vi "Choreo_Choreo_LoadTrajectoryTypeString.vi"(11 "trajectoryJsonString":string) -> (0 "Error":bool, 3 "TrajectoryType":T1)   [LabVIEW 2019, in "ChoreoLib.lvlib"]
doc: "Parse a choreo trajectory from a JSON formatted string to determine the type of trajectory, differential or swerve.. \n\nInputs: \n - trajectoryJsonString - string- The string containing the choreo trajectory. These are actually internally formatted as JSON files.\n\nOutputs:\n - TrajectoryType - enum - Type of trajectory found in the file.\n - Error out - cluster - Error cluster"
uses:
  ChoreoLib.lvlib
  ENum/Choreo_Util_TrajectoryType.ctl
panel:
  out "sampleType":string
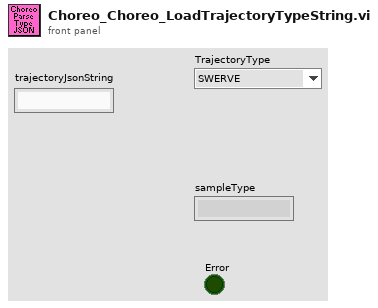
[diagram p1: front panel]
types:
  T1 = typedef "ChoreoLib.lvlib/Choreo_Util_TrajectoryType.ctl" = enum16{"SWERVE", "DIFFERENTIAL", "UNKNOWN"}
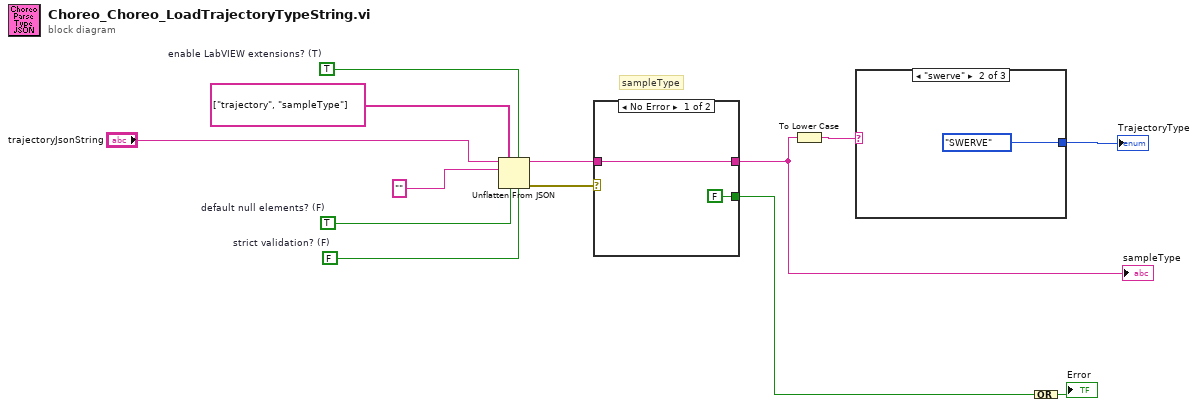
[diagram p0: block diagram]
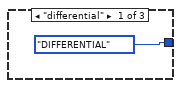
[diagram p2: hidden frame]
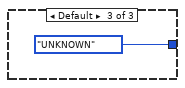
[diagram p3: hidden frame]
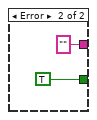
[diagram p4: hidden frame]
diagram:
  w9 = FALSE  # strict validation? (F)
  w10 = TRUE  # default null elements? (F)
  w11 = TRUE  # enable LabVIEW extensions? (T)
  # "sampleType"
  n1 = Unflatten From JSON(path=string[] ["trajectory", "sampleType"] ("path 7"), enable LabVIEW extensions? (T)=w11, JSON string="trajectoryJsonString", type and defaults="", default null elements? (F)=w10, strict validation? (F)=w9) -> (value=w12:string, error out=w13:errorcluster)  [unwired: 1 in]
  n2 = case shown="No Error" w13 {
    tunnel: w12 -> [w14 _]
    tunnel: [FALSE TRUE] -> w5
    tunnel: [w14 ""] -> w2
    frame No Error {
    }
    frame Error {
    }
  }
  "sampleType" <- w2
  n3 = To Lower Case(string=w2) -> (all lower case string=w3:string)
  n4 = case shown="\"swerve\"" w3 {
    tunnel: [Choreo_Util_TrajectoryType."DIFFERENTIAL" ("TrajectoryType") Choreo_Util_TrajectoryType."SWERVE" ("TrajectoryType") Choreo_Util_TrajectoryType."UNKNOWN" ("TrajectoryType")] -> w1
    frame "differential" {
    }
    frame "swerve" {
    }
    frame Default {
    }
  }
  "TrajectoryType" <- w1
  n5 = Compound Arithmetic op=OR(w5) -> (→"Error":bool)
